vi "UVW orientation correction.vi"(6 "(U, V, W) array in":sgl[][](array[numeric]), 7 "Relative yaw (deg)":sgl=1.0, 8 "Relative pitch (deg)":sgl, 9 "Relative roll (deg)":sgl) -> (3 "(U, V, W) array out":sgl[][](array[numeric]))   [LabVIEW 2017]
panel:
  # "PN 23/03/18"
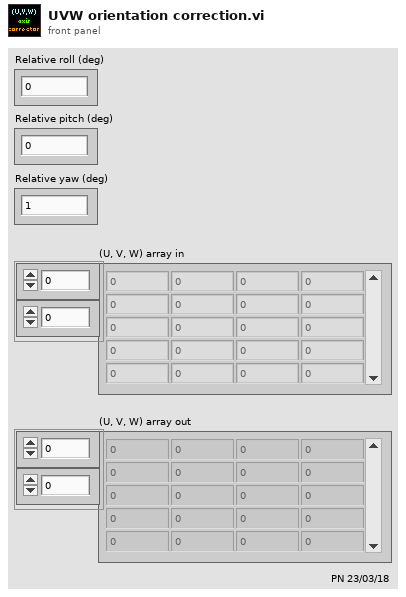
[diagram p1: front panel]
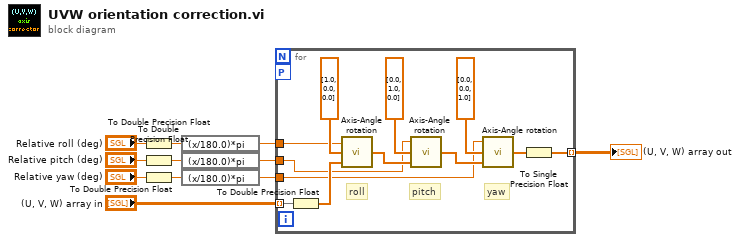
[diagram p0: block diagram]
diagram:
  n1 = To Double Precision Float(number="Relative roll (deg)") -> (double precision float=w3:dbl)
  n2 = To Double Precision Float(number="Relative pitch (deg)") -> (double precision float=w2:dbl)
  n3 = To Double Precision Float(number="Relative yaw (deg)") -> (double precision float=w1:dbl)
  n4 = expression code="(x/180.0)*pi" ("degrees to radians")(w3) -> (w6:dbl)
  n5 = expression code="(x/180.0)*pi" ("degrees to radians")(w2) -> (w5:dbl)
  n6 = expression code="(x/180.0)*pi" ("degrees to radians")(w1) -> (w4:dbl)
  n7 = for {
    tunnel: "(U, V, W) array in" -> [w23] mode=indexing
    tunnel: [w22] -> w10 mode=indexing
    workers-P: _ -> [_]
    tunnel: w6 -> [w14]
    tunnel: w5 -> [w13]
    tunnel: w4 -> [w12]
    # "yaw"
    # "pitch"
    # "roll"
    n8 = To Double Precision Float(number=w23) -> (double precision float=w19:dbl[])
    n9 = call "Axis-Angle rotation.vi"("Input vector3"=w19, "Rotation axis (UNIT vector3)"=dbl[] [1.0, 0.0, 0.0], "Rotation angle (rad)"=w14) -> ("Output vector3"=w18:dbl[])
    n10 = call "Axis-Angle rotation.vi"("Input vector3"=w18, "Rotation axis (UNIT vector3)"=dbl[] [0.0, 1.0, 0.0], "Rotation angle (rad)"=w13) -> ("Output vector3"=w17:dbl[])
    n11 = call "Axis-Angle rotation.vi"("Input vector3"=w17, "Rotation axis (UNIT vector3)"=dbl[] [0.0, 0.0, 1.0], "Rotation angle (rad)"=w12) -> ("Output vector3"=w21:dbl[])
    n12 = To Single Precision Float(number=w21) -> (single precision float=w22:sgl[])
  }
  "(U, V, W) array out" <- w10
